vi "串口测试.vi"() -> ()   [LabVIEW 2015]
uses:
  <vilib>/Instr/_visa.llb/VISA Configure Serial Port (Instr).vi
panel:
  out "字符串":string
  out "*(类型 *) &x":i64
  out "XY图":cluster{i32[], i32[]}(graph)
  out "波形图表":cluster{dbl, dbl}(graph)
  out "波形图":cluster{i32, i32, i32[]}(graph)
  in  "清空按钮":bool
  in  "暂停按钮":bool
  out "缓冲区处理后":string
  out "缓冲区字节数":u32
  out "读取缓冲区":string
  in  "停止":bool
  out "error out":errorcluster caption="错误输出"
  in  "baud rate (115200)":u32=115200 caption="波特率(115200)"
  in  "VISA resource name":refnum<visa-resource-name> caption="VISA资源名称"
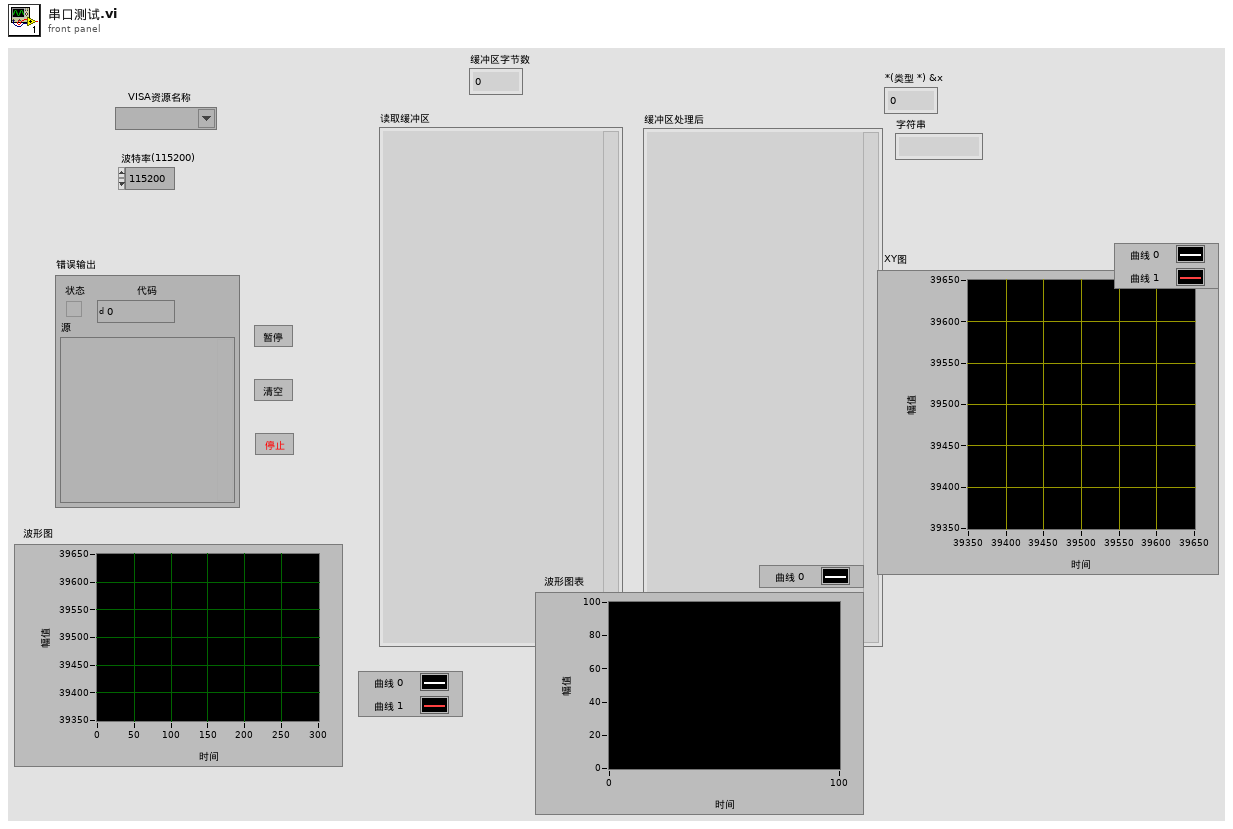
[diagram p1: front panel]
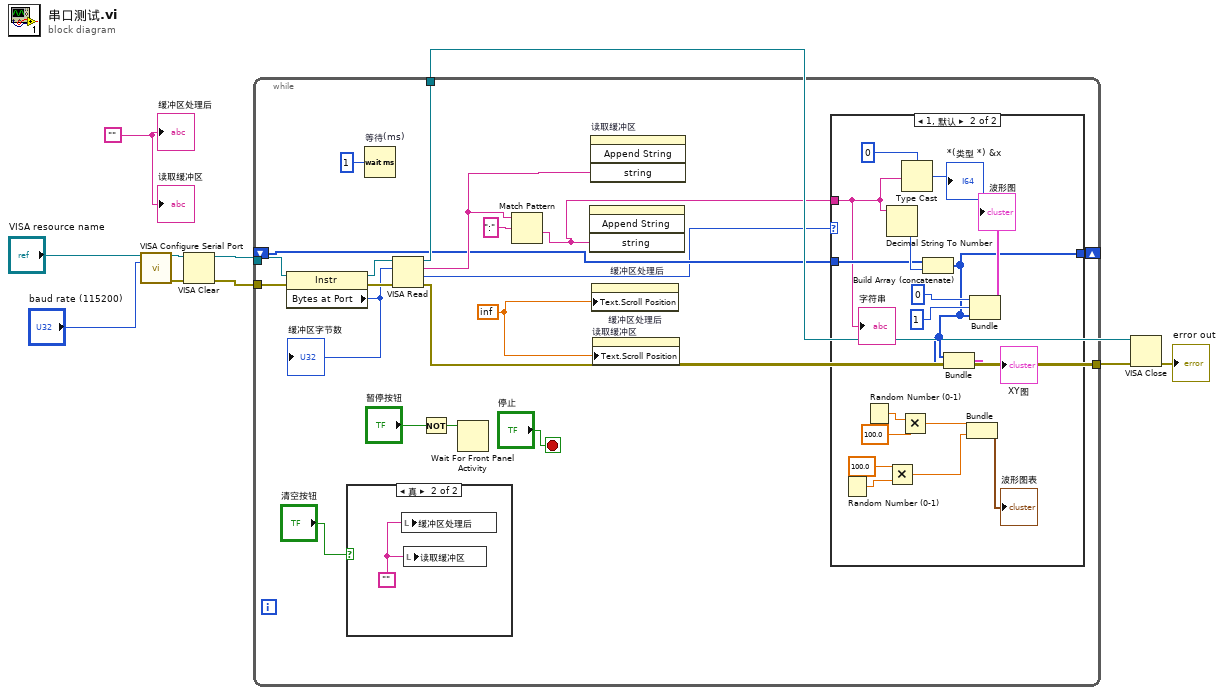
[diagram p0: block diagram]
diagram:
  w1 = ""
  n1 = call-poly "VISA Configure Serial Port"("VISA resource name"="VISA resource name", "baud rate (9600)"="baud rate (115200)") -> ("VISA resource name out"=w8:refnum<visa-resource-name>, "error out"=w6:errorcluster)  [unwired: 12 in]
  n2 = VISA Clear(VISA resource name=w8, error in (no error)=w6) -> (VISA resource name out=w7:refnum<visa-resource-name>, error out=w5:errorcluster)
  n3 = while {
    tunnel: w7 -> [w27]
    tunnel: w5 -> [w26]
    tunnel: [w22] -> w3
    tunnel: [w19] -> w2
    shift-right: [w13] -> _
    shift-left: _ -> [w14]
    stop <- "停止" stop-if-true
    w18 = inf
    n4 = property class="Instr"(reference=w27, error in=w26) -> (reference out=w25:refnum<visa-resource-name>, error out=w24:errorcluster, "Bytes at Port"=w23:u32)
    "缓冲区字节数" <- w23
    n5 = case shown="真" "清空按钮" {
      frame False {
      }
      frame True {
        w48 = ""
        n6 = local write "缓冲区处理后"(w48) -> ()
        n7 = local write "读取缓冲区"(w48) -> ()
      }
    }
    n8 = Wait (ms) "等待(ms)"(milliseconds to wait=u32 1 ("毫秒计时值")) -> ()  [unwired: 1 out]
    n9 = VISA Read(VISA resource name=w25, byte count=w23, error in (no error)=w24) -> (VISA resource name out=w19:refnum<visa-resource-name>, read buffer=w20:string, return count=w11:u32, error out=w22:errorcluster)
    n10 = Not(x="暂停按钮") -> (.not. x?=w16:bool)
    n11 = Wait For Front Panel Activity(3:w16) -> ()  [unwired: 2 in, 1 out]
    n12 = Match Pattern(string=w20, regular expression=":" ("正则表达式")) -> (after substring=w12:string)  [unwired: 1 in, 3 out]
    n13 = invoke on="缓冲区处理后" class="Str" method="Append String"("string"=w12) -> ()  [unwired: 3 in, 4 out]
    n14 = invoke on="读取缓冲区" class="Str" method="Append String"("string"=w20) -> ()  [unwired: 3 in, 4 out]
    n15 = property on="缓冲区处理后" class="Str"("Text.Scroll Position"=w18) -> ()  [unwired: 2 in, 2 out]
    n16 = property on="读取缓冲区" class="Str"("Text.Scroll Position"=w18) -> ()  [unwired: 2 in, 2 out]
    n17 = case shown="1, 默认" w11 {
      tunnel: w14 -> [w30 w46]
      tunnel: [w30 w35] -> w13
      tunnel: w12 -> [_ w31]
      frame 0 {
      }
      frame 1, Default {
        n18 = Random Number (0-1)() -> (number: 0 to 1=w42:dbl)
        n19 = Random Number (0-1)() -> (number: 0 to 1=w39:dbl)
        n20 = Decimal String To Number(string=w31) -> (number=w47:i32)  [unwired: 2 in, 1 out]
        n21 = Multiply(x=100.0, y=w42) -> (x*y=w40:dbl)
        n22 = Multiply(x=w39, y=100.0) -> (x*y=w38:dbl)
        n23 = Type Cast(type=i8 0, x=w31) -> (*(type *) &x=→"*(类型 *) &x":i8)
        n24 = Build Array (concatenate)(w46, w47) -> (w35:i32[])
        n25 = Bundle(w35, w35) -> (→"XY图":cluster{i32[], i32[]})  [unwired: 1 in]
        n26 = Bundle(w38, w40) -> (→"波形图表":cluster{dbl, dbl})  [unwired: 1 in]
        n27 = Bundle(0, 1, w35) -> (→"波形图":cluster{i32, i32, i32[]})  [unwired: 1 in]
        "字符串" <- w31
      }
    }
  }
  n28 = VISA Close(VISA resource name=w2, error in (no error)=w3) -> (error out=→"error out":errorcluster)
  "读取缓冲区" <- w1
  "缓冲区处理后" <- w1
